vi "Get Board ID.vi"(8 "error in":errorcluster, 11 "custom device ref":T1 format="%.0x") -> (0 "error out":errorcluster, 2 "Board ID":i32, 3 "custom device ref out":T1 format="%.0x")   [LabVIEW 2020, in "AIM ARINC 664 Scripting.lvlib"]
uses:
  AIM ARINC 664 Scripting.lvlib
  <vilib>/NI VeriStand/Custom Device API/Custom Device Item Ref.ctl
  Constants.vi
  <vilib>/NI VeriStand/Custom Device API/Custom Device API.lvlib
  <vilib>/NI VeriStand/Custom Device API/Get Item Property (I32).vi
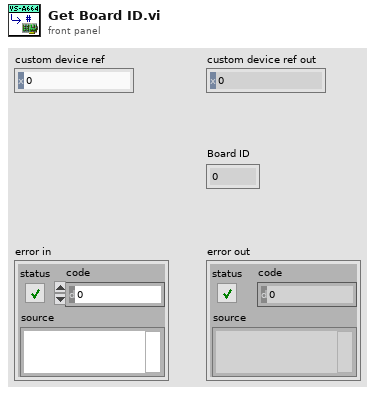
[diagram p1: front panel]
types:
  T1 = typedef "Custom Device API.lvlib/Custom Device Item Ref.ctl" = u64
  T2 = typedef "AIM ARINC 664 Import.lvlib/board_setup.ctl" = cluster{"boardId":u32, "portSpeed":u32, "portConfig":u32}
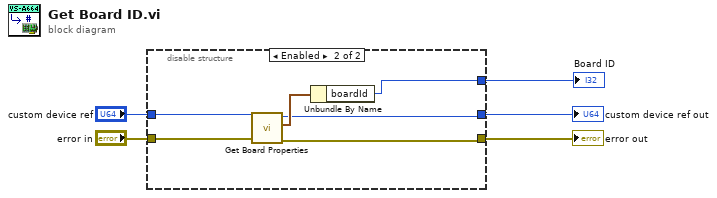
[diagram p0: block diagram]
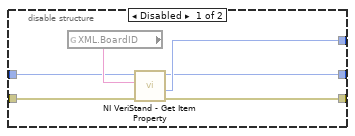
[diagram p2: hidden frame]
diagram:
  n1 = disable-structure shown="Enabled" {
    disable-tunnel: "custom device ref" -> [w10 w17]
    disable-tunnel: "error in" -> [w9 w16]
    disable-tunnel: [w8 w14] -> w3
    disable-tunnel: [w7 w12] -> w2
    disable-tunnel: [w6 w13] -> w1
    frame Disabled {
      n2 = global read "Constants.vi" "XML.BoardID"() -> (w11:string)
      n3 = call-poly <vilib>:"NI VeriStand - Get Item Property.vi"("error in (no error)"=w9, "Property Name"=w11, "Item Ref in"=w10) -> ("error out"=w7:errorcluster, "Value"=w8:i32, "Item Ref out"=w6:T1)  [unwired: 5 in, 1 out]
    }
    frame Enabled {
      n4 = call "Get Board Properties.vi"("error in"=w16, "custom device ref"=w17) -> ("error out"=w12:errorcluster, "board properties out"=w15:T2, "custom device ref out"=w13:T1)  [unwired: 7 in]
      n5 = Unbundle By Name(w15) -> ("boardId"=w14:u32)
    }
  }
  "custom device ref out" <- w1
  "error out" <- w2
  "Board ID" <- w3
